vi "Version 1_Read Power-up Settings.vi"(7 "Address (A)":string="A", 8 "error in":errorcluster, 11 "VISA Session In":refnum<visa-resource-name>="Alicat") -> (0 "error out":errorcluster, 1 "Power-up":T1={"Serial/Local Setpoint"=enum."Save", "FP Buttons"=enum."Unlocked", "Valve Hard Zero"=enum."On zero setpoint", "Initial Screen"=enum."Main", "Gas Select"=enum."Save", "Control Range"=enum."Unknown", "Tare Delay"=nan}, 3 "VISA Session Out":refnum<visa-resource-name>)   [LabVIEW 2014]
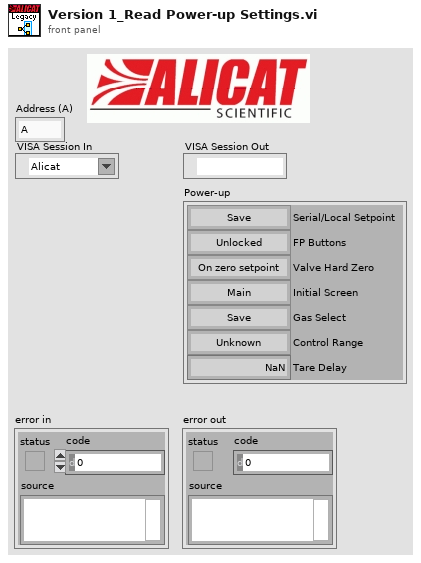
[diagram p1: front panel]
types:
  T1 = cluster{"Serial/Local Setpoint":enum8{"Don't Save", "Save"}, "FP Buttons":enum8{"Unlocked", "Locked"}, "Valve Hard Zero":enum16{"On zero setpoint", "Startup only"}, "Initial Screen":enum16{"Main", "Totalizer"}, "Gas Select":enum8{"Don't Save", "Save"}, "Control Range":enum16{"Normal", "Invert", "Bipolar", "Unknown"}, "Tare Delay":dbl}
  T2 = cluster{"Serial/Local Setpoint":enum8{"Don't Save", "Save"}, "FP Buttons":enum8{"Unlocked", "Locked"}, "Valve Hard Zero":enum16{"On zero setpoint", "Startup only"}, "Initial Screen":enum16{"Main", "Totalizer"}, "Gas Select":enum8{"Don't Save", "Save"}, "Tare Delay":dbl, "Control Range":enum16{"Normal", "Inverted", "Bidirectional", "Unknown"}}
  T3 = enum16{"Normal", "Inverted", "Bidirectional", "Unknown"}
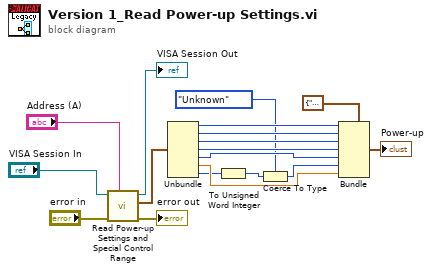
[diagram p0: block diagram]
diagram:
  n1 = call "Read Power-up Settings and Special Control Range.vi"("Unit ID (A)"="Address (A)", "error in"="error in", "VISA Session In"="VISA Session In") -> ("error out"=→"error out":errorcluster, "Power-up settings & special control range"=w13:T2, "VISA Session Out"=→"VISA Session Out":refnum<visa-resource-name>)  [unwired: 6 in]
  n2 = Unbundle(w13) -> ("Serial/Local Setpoint"=w10:enum8{"Don't Save", "Save"}, "FP Buttons"=w9:enum8{"Unlocked", "Locked"}, "Valve Hard Zero"=w7:enum16{"On zero setpoint", "Startup only"}, "Initial Screen"=w8:enum16{"Main", "Totalizer"}, "Gas Select"=w6:enum8{"Don't Save", "Save"}, "Tare Delay"=w5:dbl, "Control Range"=w1:T3)
  n3 = To Unsigned Word Integer(number=w1) -> (unsigned 16bit integer=w2:u16)
  n4 = Coerce To Type(0:w2, 1:enum16{"Normal", "Invert", "Bipolar", "Unknown"}."Unknown" ("Control Range")) -> (2:w3:enum16{"Normal", "Invert", "Bipolar", "Unknown"})
  n5 = Bundle(cluster=T1 {"Serial/Local Setpoint"=enum."Save", "FP Buttons"=enum."Unlocked", "Valve Hard Zero"=enum."On zero setpoint", "Initial Screen"=enum."Main", "Gas Select"=enum."Save", "Control Range"=enum."Unknown", "Tare Delay"=nan} ("Power-up"), "Serial/Local Setpoint"=w10, "FP Buttons"=w9, "Valve Hard Zero"=w7, "Initial Screen"=w8, "Gas Select"=w6, "Control Range"=w3, "Tare Delay"=w5) -> (→"Power-up":T1)
